vi "ExampleMeasurementServer.vi"() -> ()   [LabVIEW 2019]
uses:
  VIs/QueryServer_FourProbeRawData.ctl
  VIs/QueryServer_ErrorOutData.ctl
  VIs/labview-grpc-query-server.lvlib
panel:
  in  "Server Key File (.key)":path
  in  "Server Certificate File (.crt)":path
  in  "stop":bool
  in  "Server Address":string="0.0.0.0:50051"
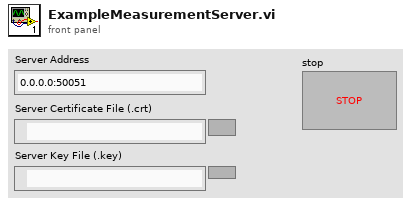
[diagram p1: front panel]
types:
  T1 = typedef "labview-grpc-query-server.lvlib/QueryServer_gRPCid.ctl" = u64
  T2 = cluster{"QueryServer_Invoke":refnum<user-event>, "QueryServer_Query":refnum<user-event>, "QueryServer_Register":refnum<user-event>, "QueryServer_FourProbeMeasurement":refnum<user-event>, "gRPCid":T1}
  T3 = typedef "labview-grpc-query-server.lvlib/QueryServer_ErrorOutData.ctl" = cluster{"ErrorCode":i32, "ErrorMessage":string}
  T4 = typedef "labview-grpc-query-server.lvlib/QueryServer_FourProbeRawData.ctl" = cluster{"Positive Voltage":sgl, "Positive Current":sgl, "Negative Voltage":sgl, "Negative Current":sgl, "Impedance":sgl, "ErrorOutData":T3}
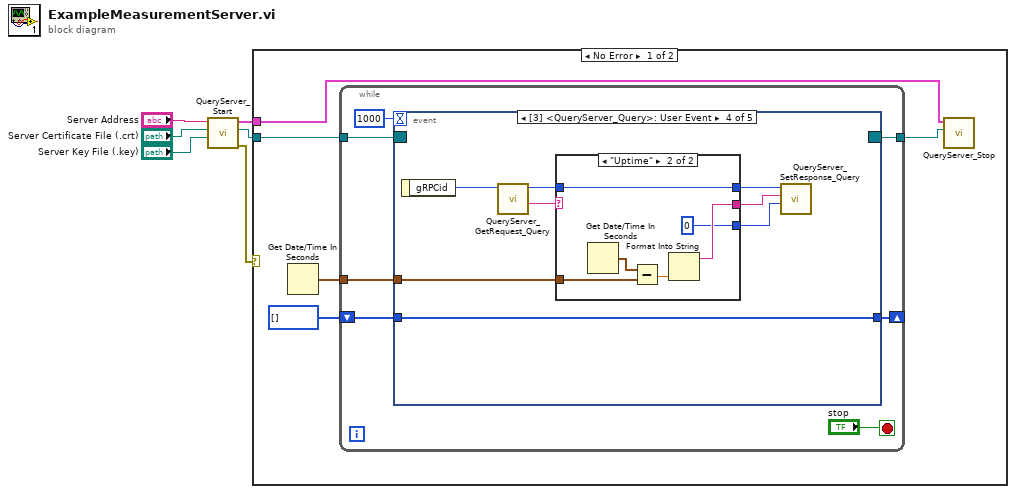
[diagram p0: block diagram]
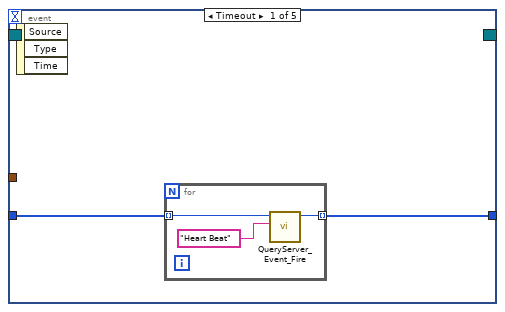
[diagram p2: hidden frame]
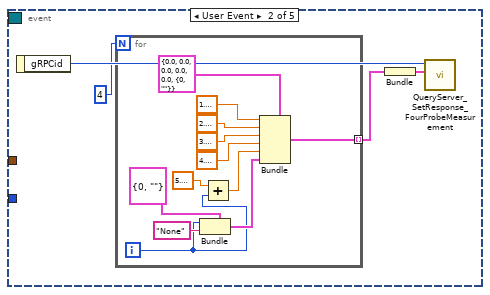
[diagram p3: hidden frame]
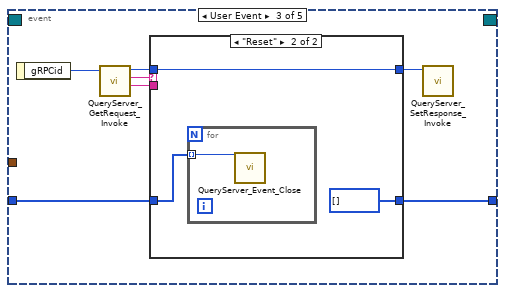
[diagram p4: hidden frame]
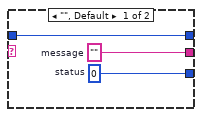
[diagram p6: hidden frame]
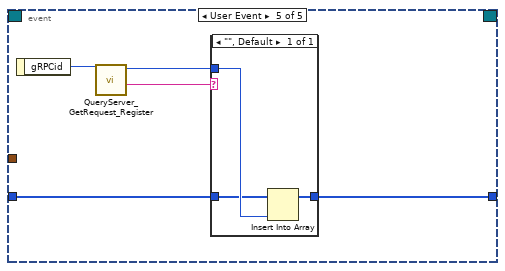
[diagram p7: hidden frame]
diagram:
  n1 = call "QueryServer_Start.vi"("Server Key File (.key)"="Server Key File (.key)", "Server Certificate File (.crt)"="Server Certificate File (.crt)", "Server Address"="Server Address") -> ("error out"=w2:errorcluster, "Event Registration Refnum"=w1:refnum<event-registration>, "Server Information"=w5:T2)  [unwired: 5 in]
  n2 = case shown="No Error" w2 {
    tunnel: w5 -> [w9 _]
    tunnel: w1 -> [w8 _]
    frame No Error {
      n3 = Get Date/Time In Seconds() -> (seconds since 1Jan1904=w11:timestamp)
      n4 = while {
        tunnel: [w17] -> w7
        tunnel: w11 -> [w16]
        shift-right: [w14] -> _
        shift-left: u64[] [] -> [w13]
        tunnel: w8 -> [w12]
        stop <- "stop" stop-if-true
        n5 = event shown="[3] <QueryServer_Query>: User Event" {
          selector: w12 -> [_ _ _ _ _]
          dyn-events: [_ _ _ _ _] -> w17
          timeout: 1000 -> [_ _ _ _ _]
          tunnel: w16 -> [_ _ _ w55 _]
          tunnel: [w20 _ w40 w54 w72] -> w14
          tunnel: w13 -> [w19 _ w41 w54 w71]
          event Timeout {
            n6 = event-data() -> ()  [unwired: 1 in, 3 out]
            n7 = for {
              tunnel: w19 -> [w23] mode=indexing
              tunnel: [w21] -> w20 mode=indexing
              n8 = call "QueryServer_Event_Fire.vi"("eventdata"="Heart Beat", "gRPCid"=w23) -> ("gRPCid out"=w21:T1)  [unwired: 8 in, 1 out]
            }
          }
          event User Event {
            n9 = event-data() -> ("gRPCid"=w27:T1)  [unwired: 1 in]
            n10 = for {
              N: 4 -> [_]
              tunnel: [w37] -> w25 mode=indexing
              i -> [w29]
              n11 = Bundle(cluster=T3 {"ErrorCode"=0, "ErrorMessage"=""} ("ErrorOutData"), "ErrorCode"=w29, "ErrorMessage"="None") -> (w38:T3)
              n12 = Add(x=sgl 5.1 ("Positive Voltage"), y=w29) -> (x+y=w28:sgl)
              n13 = Bundle(cluster=T4 {"Positive Voltage"=0.0, "Positive Current"=0.0, "Negative Voltage"=0.0, "Negative Current"=0.0, "Impedance"=0.0, "ErrorOutData"={"ErrorCode"=0, "ErrorMessage"=""}} ("FourProbeRawData"), "Positive Voltage"=sgl 1.1, "Positive Current"=sgl 2.1 ("Positive Voltage"), "Negative Voltage"=sgl 3.1 ("Positive Voltage"), "Negative Current"=sgl 4.1 ("Positive Voltage"), "Impedance"=w28, "ErrorOutData"=w38) -> (w37:T4)
            }
            n14 = Bundle(w25) -> (w24:cluster{T4[]})  [unwired: 1 in]
            n15 = call "QueryServer_SetResponse_FourProbeMeasurement.vi"("gRPCid"=w27, "FourProbeResponse"=w24) -> ()  [unwired: 8 in, 1 out]
          }
          event User Event {
            n16 = event-data() -> ("gRPCid"=w46:T1)  [unwired: 1 in]
            n17 = call "QueryServer_GetRequest_Invoke.vi"("gRPCid"=w46) -> ("parameter"=w42:string, "command"=w45:string, "gRPCid out"=w44:T1)  [unwired: 5 in, 1 out]
            n18 = case shown="\"Reset\"" w45 {
              tunnel: w44 -> [w48 w49]
              tunnel: [w48 w49] -> w43
              tunnel: w42 -> [_ _]
              tunnel: w41 -> [w47 w51]
              tunnel: [w47 u64[] []] -> w40
              frame "", Default {
              }
              frame "Reset" {
                n19 = for {
                  tunnel: w51 -> [w52] mode=indexing
                  n20 = call "QueryServer_Event_Close.vi"("gRPCid"=w52) -> ()  [unwired: 9 in, 1 out]
                }
              }
            }
            n21 = call "QueryServer_SetResponse_Invoke.vi"("gRPCid"=w43) -> ()  [unwired: 9 in, 1 out]
          }
          event User Event {
            n22 = event-data() -> ("gRPCid"=w60:T1)  [unwired: 1 in]
            n23 = call "QueryServer_GetRequest_Query.vi"("gRPCid"=w60) -> ("gRPCid out"=w59:T1, "query"=w53:string)  [unwired: 7 in, 1 out]
            n24 = case shown="\"Uptime\"" w53 {
              tunnel: w59 -> [w63 w65]
              tunnel: [w63 w65] -> w58
              tunnel: [w62 w66] -> w57
              tunnel: [w61 0 ("status")] -> w56
              tunnel: w55 -> [_ w68]
              frame "", Default {
                w61 = 0  # status
                w62 = ""  # message
              }
              frame "Uptime" {
                n25 = Get Date/Time In Seconds() -> (seconds since 1Jan1904=w69:timestamp)
                n26 = Subtract(x=w69, y=w68) -> (x-y=w67:dbl)
                n27 = Format Into String(w67) -> (resulting string=w66:string)  [unwired: 3 in, 1 out]
              }
            }
            n28 = call "QueryServer_SetResponse_Query.vi"("gRPCid"=w58, "message"=w57, "status"=w56) -> ()  [unwired: 7 in, 1 out]
          }
          event User Event {
            n29 = event-data() -> ("gRPCid"=w74:T1)  [unwired: 1 in]
            n30 = call "QueryServer_GetRequest_Register.vi"("gRPCid"=w74) -> ("gRPCid out"=w73:T1, "eventname"=w70:string)  [unwired: 7 in, 1 out]
            n31 = case shown="\"\", Default" w70 {
              tunnel: w73 -> [w77]
              tunnel: [w76] -> w72
              tunnel: w71 -> [w75]
              frame "", Default {
                n32 = Insert Into Array(array=w75, new element=w77) -> (w76:T1[])  [unwired: 1 in]
              }
            }
          }
        }
      }
      n33 = call "QueryServer_Stop.vi"("Server Information"=w9, "Event Registration Refnum"=w7) -> ()  [unwired: 8 in, 1 out]
    }
    frame Error {
    }
  }
